vi "AOselector.vi"(8 "I/O element":T1(ring), 11 "value":i16) -> ()   [LabVIEW 2014]
uses:
  <vilib>/rvi/eio/common/nirviEmuTemplateMethod_errors.vi
  <vilib>/eio/EIONode/EIONode.xnode
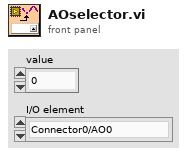
[diagram p1: front panel]
types:
  T1 = enum16{"Connector0/AO0", "Connector0/AO1", "Connector0/AO2", "Connector0/AO3", "Connector0/AO4", "Connector0/AO5", "Connector0/AO6", "Connector0/AO7"}
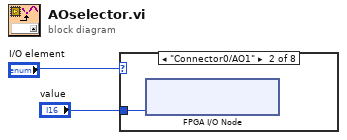
[diagram p0: block diagram]
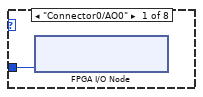
[diagram p2: hidden frame]
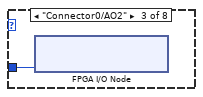
[diagram p3: hidden frame]
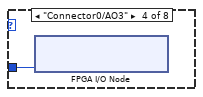
[diagram p4: hidden frame]
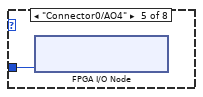
[diagram p5: hidden frame]
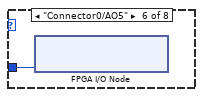
[diagram p6: hidden frame]
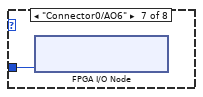
[diagram p7: hidden frame]
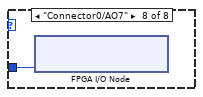
[diagram p8: hidden frame]
diagram:
  n1 = case shown="\"Connector0/AO1\"" "I/O element" {
    tunnel: "value" -> [w3 w4 w5 w6 w7 w8 w9 w10]
    frame "Connector0/AO0" {
      n2 = xnode "FPGA I/O Node"("Connector0/AO0"=w3) -> ()  [unwired: 1 in, 1 out]
    }
    frame "Connector0/AO1" {
      n3 = xnode "FPGA I/O Node"("Connector0/AO1"=w4) -> ()  [unwired: 1 in, 1 out]
    }
    frame "Connector0/AO2" {
      n4 = xnode "FPGA I/O Node"("Connector0/AO2"=w5) -> ()  [unwired: 1 in, 1 out]
    }
    frame "Connector0/AO3" {
      n5 = xnode "FPGA I/O Node"("Connector0/AO3"=w6) -> ()  [unwired: 1 in, 1 out]
    }
    frame "Connector0/AO4" {
      n6 = xnode "FPGA I/O Node"("Connector0/AO4"=w7) -> ()  [unwired: 1 in, 1 out]
    }
    frame "Connector0/AO5" {
      n7 = xnode "FPGA I/O Node"("Connector0/AO5"=w8) -> ()  [unwired: 1 in, 1 out]
    }
    frame "Connector0/AO6" {
      n8 = xnode "FPGA I/O Node"("Connector0/AO6"=w9) -> ()  [unwired: 1 in, 1 out]
    }
    frame "Connector0/AO7" {
      n9 = xnode "FPGA I/O Node"("Connector0/AO7"=w10) -> ()  [unwired: 1 in, 1 out]
    }
  }
